vi "Update Record Time.vi"(8 "error in":errorcluster, 11 "Instruments in":refnum<class "Instruments.lvclass">) -> (0 "error out":errorcluster, 2 "Data Pad Count":i32, 3 "Instruments out":refnum<class "Instruments.lvclass">)   [LabVIEW 2019, in "Instruments.lvlib" / "Instruments.lvclass"]
uses:
  Instruments.lvclass
  Instruments.lvclass/Instruments.ctl
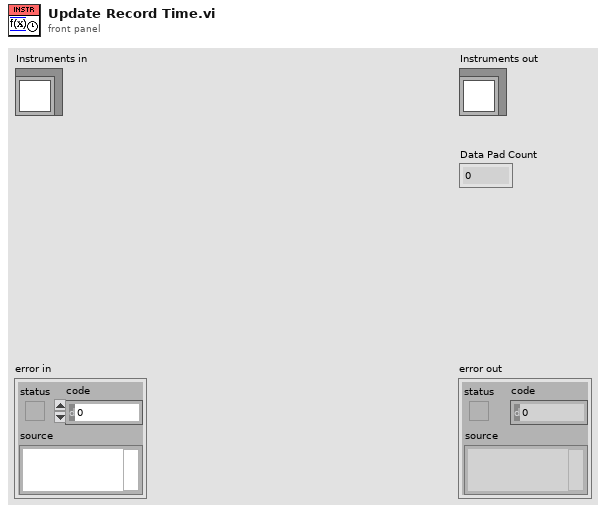
[diagram p1: front panel]
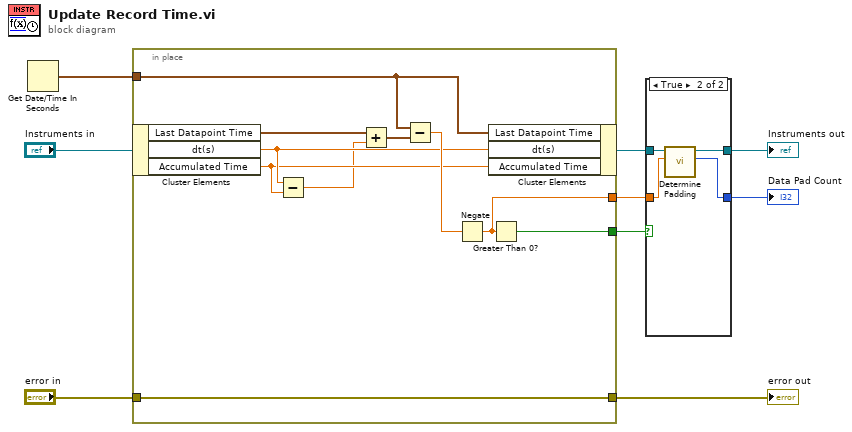
[diagram p0: block diagram]
diagram:
  n1 = Get Date/Time In Seconds() -> (seconds since 1Jan1904=w8:timestamp)
  n2 = in-place {
    in-place-border: w8 -> [w17]
    in-place-border: "error in" -> [w16]
    in-place-border: [w16] -> w6
    in-place-border: [w15] -> w5
    in-place-border: [w13] -> w2
    n3 = in-place-cluster #1("Instruments in") -> ("Last Datapoint Time"=w19:timestamp, "dt(s)"=w12:dbl, "Accumulated Time"=w11:dbl)
    n4 = Subtract(x=w12, y=w11) -> (x-y=w10:dbl)
    n5 = Add(x=w19, y=w10) -> (x+y=w18:timestamp)
    n6 = Subtract(x=w17, y=w18) -> (x-y=w14:dbl)
    n7 = Negate(x=w14) -> (-x=w13:dbl)
    n8 = in-place-cluster #1("Last Datapoint Time"=w17, "dt(s)"=w12, "Accumulated Time"=w11) -> (w4:refnum<class "Instruments.lvclass">)
    n9 = Greater Than 0?(x=w13) -> (x > 0?=w15:bool)
  }
  "error out" <- w6
  n10 = case shown="True" w5 {
    tunnel: w4 -> [w20 w24]
    tunnel: [w20 w23] -> w3
    tunnel: w2 -> [_ w22]
    tunnel: [_ w21] -> w1
    frame False {
    }
    frame True {
      n11 = call "Determine Padding.vi"("Actual dt"=w22, "Instruments in"=w24) -> ("Data Pad Count"=w21:i32, "Instruments out"=w23:refnum<class "Instruments.lvclass">)  [unwired: 7 in, 1 out]
    }
  }
  "Instruments out" <- w3
  "Data Pad Count" <- w1
